vi "Instantaneous DC Setup.vi"   [LabVIEW 2010]
uses:
  <vilib>/DAQmx/configure/timing.llb/DAQmx Timing (Sample Clock).vi
  <vilib>/DAQmx/configure/timing.llb/DAQmx Timing (Implicit).vi
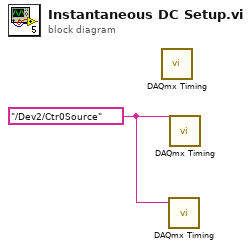
[diagram p0: block diagram]
diagram:
  w1 = tag "/Dev2/Ctr0Source" ("source")
  n1 = call-poly <vilib>:"DAQmx Timing.vi"() -> ()  [unwired: 14 in, 2 out]
  n2 = call-poly <vilib>:"DAQmx Timing.vi"("source"=w1) -> ()  [unwired: 13 in, 2 out]
  n3 = call-poly <vilib>:"DAQmx Timing.vi"("source"=w1) -> ()  [unwired: 13 in, 2 out]
